vi "Write Siemens Digital Energy Meter.vi"(8 "error in (no error)":errorcluster, 10 "Siemens Digital Energy Meter":T1 {"Measurement(s)" items=["kWh System"=4000, "kVARh System"=4007, "kVAh System"=4010, "kVA System"=4012, "Volts L1 to L2"=4018, "Volts L2 to L3"=4019, "Volts L1 to L2"=4020, "Line Frequency"=4021, "kW L1"=4028, "kW L2"=4029, "kW L3"=4030, "kVAR L1"=4037, "kVAR L2"=4038, "kVAR L3"=4039, "kVA L1"=4046, "kVA L2"=4047, "kVA L3"=4048, "Apparent PF L1"=4052, "Apparent PF L2"=4053, "Apparent PF L3"=4054, "Amps L1"=4055, "Amps L2"=4056, "Amps L3"=4057, "Volts L1 to Neutral"=4058, "Volts L2 to Neutral"=4059, "Volts L3 to Neutral"=4060, "Firmware Major Revision"=4068, "Firmware Minor Revision "=4069, "Model Number "=4200, "Serial Number"=4205, "Hardware ID"=4510]}, 11 "SiemensDigitalEnergyMeter in":refnum<class "SiemensDigitalEnergyMeter.lvclass">) -> (0 "error out":errorcluster, 3 "SiemensDigitalEnergyMeter out":refnum<class "SiemensDigitalEnergyMeter.lvclass">)   [LabVIEW 2018, in "SensorPlugins.lvlib" / "SiemensDigitalEnergyMeter.lvclass"]
uses:
  SiemensDigitalEnergyMeter.lvclass
  TypeDefinitions/SiemensDigitalEnergyMeterControls.ctl
  SiemensDigitalEnergyMeter.lvclass/SiemensDigitalEnergyMeter.ctl
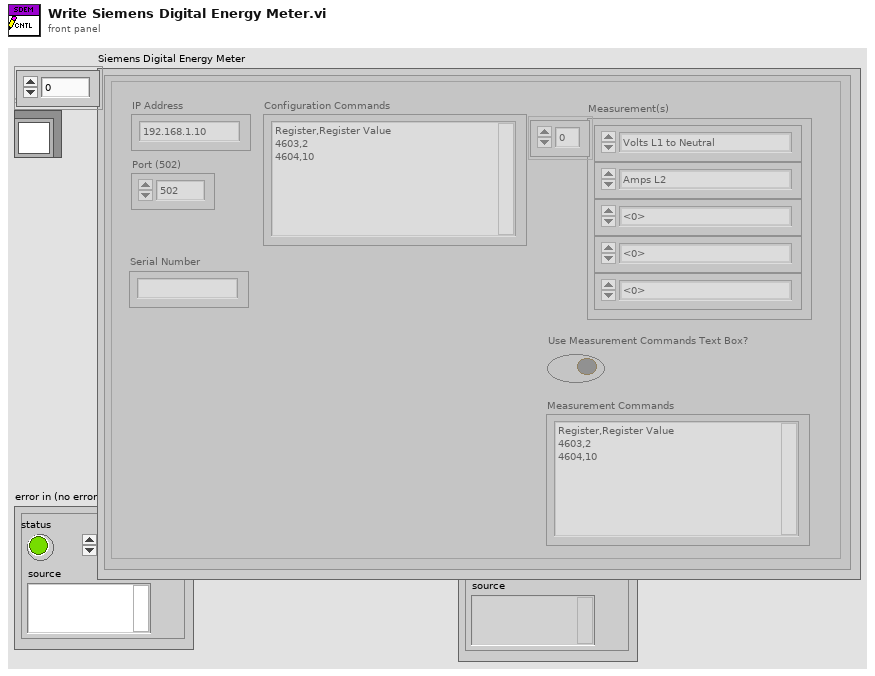
[diagram p1: front panel]
types:
  T1 = typedef "SensorPlugins.lvlib/SiemensDigitalEnergyMeter.lvclass/SiemensDigitalEnergyMeterControls.ctl" = cluster{"Measurement(s)":u16[], "IP Address":string, "Port (502)":u16, "Configuration Commands":string, "Use Measurement Commands Text Box?":bool, "Measurement Commands":string, "Connected?":bool, "Serial Number":string}[]
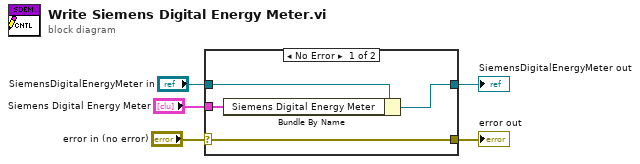
[diagram p0: block diagram]
diagram:
  n1 = case shown="No Error" "error in (no error)" {
    selector: "error in (no error)" -> [w9 w10]
    tunnel: [w9 w10] -> w4
    tunnel: [w7 w11] -> w2
    tunnel: "SiemensDigitalEnergyMeter in" -> [w8 w11]
    tunnel: "Siemens Digital Energy Meter" -> [w6 _]
    frame No Error {
      n2 = Bundle By Name(cluster=w8, "Siemens Digital Energy Meter"=w6) -> (w7:refnum<class "SiemensDigitalEnergyMeter.lvclass">)
    }
    frame Error {
    }
  }
  "error out" <- w4
  "SiemensDigitalEnergyMeter out" <- w2
